vi "2.vi"() -> ()   [LabVIEW 2015]
panel:
  out "result":dbl
  in  "numeric 2":dbl
  in  "numeric":dbl
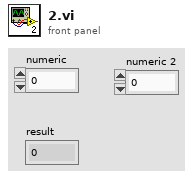
[diagram p1: front panel]
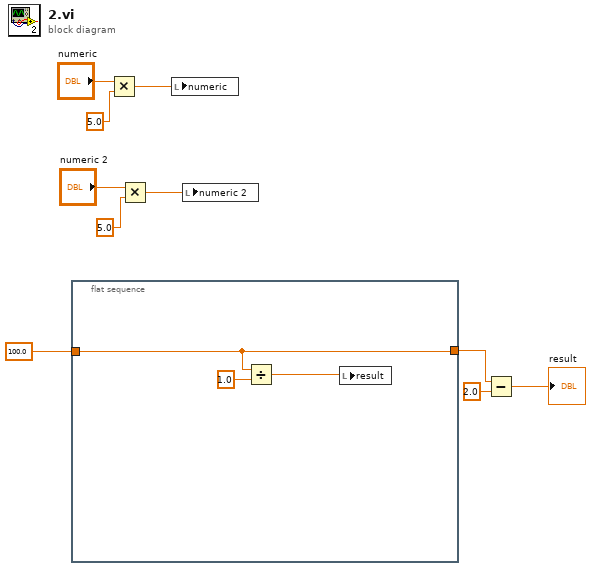
[diagram p0: block diagram]
diagram:
  n1 = flat-sequence {
    tunnel: 100.0 -> [w11]
    tunnel: [w11] -> w2
    frame #0 {
      n2 = Divide(x=w11, y=1.0) -> (x/y=w12:dbl)
      n3 = local write "result"(w12) -> ()
    }
  }
  n4 = Multiply(x="numeric", y=5.0) -> (x*y=w8:dbl)
  n5 = Multiply(x="numeric 2", y=5.0) -> (x*y=w6:dbl)
  n6 = local write "numeric"(w8) -> ()
  n7 = local write "numeric 2"(w6) -> ()
  n8 = Subtract(x=w2, y=2.0) -> (x-y=→"result":dbl)
